vi "5Decembre2016.vi"() -> ()   [LabVIEW 2014]
panel:
  out "Array":string[](array[string])
  out "Partie 1":string[](array[string])
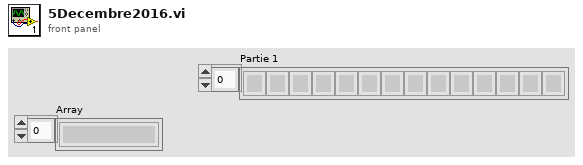
[diagram p1: front panel]
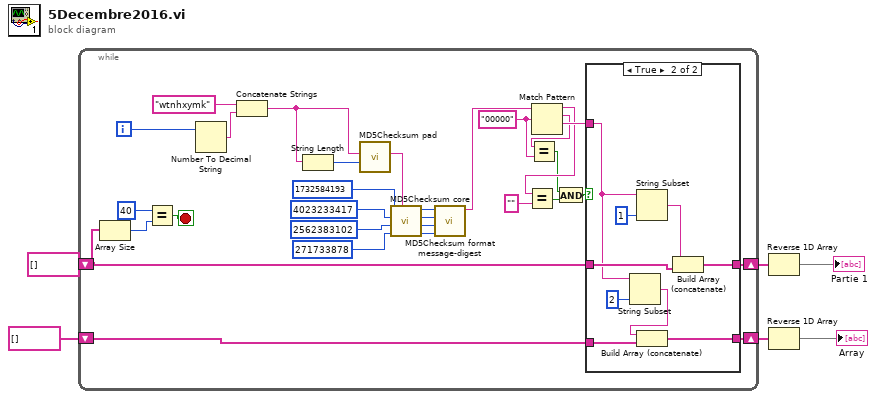
[diagram p0: block diagram]
diagram:
  n1 = while {
    shift-right: [w32] -> w6
    shift-left: string[] [] -> [w31]
    shift-right: [w8] -> w1
    shift-left: string[] [] -> [w7]
    i -> [w9]
    stop <- w36 stop-if-true
    w34 = "00000" ("regular expression")
    n2 = Array Size(array=w31) -> (size(s)=w24:i32)
    n3 = Equal?(x=40, y=w24) -> (x = y?=w36:bool)
    n4 = Number To Decimal String(number=w9) -> (decimal integer string=w22:string)  [unwired: 1 in]
    n5 = Concatenate Strings("wtnhxymk", w22) -> (w10:string)
    n6 = String Length(string=w10) -> (length=w11:i32)
    n7 = call <vilib>:"MD5Checksum pad.vi"("Message String Length (bytes)"=w11, "Last Part of Message String"=w10) -> ("Padding"=w21:string)  [unwired: 9 in]
    n8 = call <vilib>:"MD5Checksum core.vi"("Input String"=w21, "s4 in"=u32 271733878 ("s4"), "s3 in"=u32 2562383102 ("s3"), "s2 in"=u32 4023233417 ("s2"), "s1 in"=u32 1732584193 ("s1")) -> ("s4 out"=w16:u32, "s3 out"=w15:u32, "s2 out"=w14:u32, "s1 out"=w13:u32)  [unwired: 3 in]
    n9 = call <vilib>:"MD5Checksum format message-digest.vi"("s4"=w16, "s3"=w15, "s2"=w14, "s1"=w13) -> ("MD5 message-digest"=w12:string)  [unwired: 7 in]
    n10 = Match Pattern(string=w12, regular expression=w34) -> (before substring=w29:string, match substring=w33:string, after substring=w35:string)  [unwired: 1 in, 1 out]
    n11 = Equal?(x=w29, y="") -> (x = y?=w26:bool)
    n12 = Equal?(x=w33, y=w34) -> (x = y?=w27:bool)
    n13 = And(x=w27, y=w26) -> (x .and. y?=w25:bool)
    n14 = case shown="True" w25 {
      tunnel: w35 -> [_ w42]
      tunnel: w31 -> [w38 w46]
      tunnel: [w38 w47] -> w32
      tunnel: [w37 w43] -> w8
      tunnel: w7 -> [w37 w41]
      frame False {
      }
      frame True {
        n15 = String Subset(string=w42, length (rest)=2 ("length (rest)")) -> (substring=w39:string)  [unwired: 1 in]
        n16 = String Subset(string=w42, length (rest)=1 ("length (rest)")) -> (substring=w45:string)  [unwired: 1 in]
        n17 = Build Array (concatenate)(w39, w41) -> (w43:string[])
        n18 = Build Array (concatenate)(w45, w46) -> (w47:string[])
      }
    }
  }
  n19 = Reverse 1D Array(array=w6) -> (reversed array=→"Partie 1":string[])
  n20 = Reverse 1D Array(array=w1) -> (reversed array=→"Array":string[])
